vi "PSK_Mod_Transmit_test.vi"() -> ()   [LabVIEW 2014]
uses:
  <vilib>/addons/Modulation/Digital/General/MT Generate Bits (Galois, PN Order).vi
  <vilib>/addons/Modulation/Digital/Support/Common/Validators/mod_Generate Bits Validate.vi
  <vilib>/addons/Modulation/Analog/support/mod_Set Error Source.vi
  <vilib>/addons/Modulation/Digital/General/MT Generate PSK System Parameters(M).vi
  <vilib>/addons/Modulation/Digital/Support/Common/Validators/mod_Generate Filter Coefficients Validate.vi
  <vilib>/addons/Modulation/Digital/General/subVIs/mod_Generate Filter Coefficients.vi
  <vilib>/addons/Modulation/Digital/General/subVIs/mod_Generate Bits PN Sequence.vi
  <vilib>/addons/Modulation/Digital/General/MT Generate PSK Synchronization Parameters (bit array).vi
  <vilib>/addons/Modulation/Digital/General/MT Generate Bits (User Defined).vi
  <instrlib>/niUSRP/niUSRP Write Tx Data (CDB Cluster).vi
  <vilib>/addons/Modulation/niDMT.lvlib
  <vilib>/addons/Modulation/niAMT.lvlib
panel:
  out "Before demod&compensation":waveform(dbl)(graph)
  in  "stop":bool
  in  "error in (no error)":errorcluster
  out "error out":errorcluster
  in  "USRP IP address":refnum<k15>="192.168.10.1"
  in  "Tx Parameters":T1={"Tx IQ Sampling\nRate [s/sec]"=400000.0, "Tx Frequency [Hz]"=5795000000.0, "Tx Gain [dB]"=0.0, "Tx Antenna"="TX1"} {"Tx Gain [dB]" format="%#.6p"; "Tx Frequency [Hz]" format="%#.6p"; "Tx IQ Sampling\nRate [s/sec]" format="%#.6p"}
  out "Actual Tx Parameters":T1={"Tx IQ Sampling\nRate [s/sec]"=400000.0, "Tx Frequency [Hz]"=915000000.0, "Tx Gain [dB]"=0.0, "Tx Antenna"="TX1"} {"Tx Gain [dB]" format="%#.6p"; "Tx Frequency [Hz]" format="%#.6p"; "Tx IQ Sampling\nRate [s/sec]" format="%#.6p"}
  in  "user base bit pattern":i8[](array[numeric]) caption="Input bit stream"
  out "bits sent":i32
  out "Constellation Graph":T2(graph) caption="Tx Signal Constellation"
  out "input bit stream":i8[](array[numeric]) caption="input package"
  in  "filter parameters":T3={"Alpha"=0.5, "Filter Length"=6, "TX Filter"=enum."Root Raised Cos"} {"Alpha" format="%.2f"}
  in  "QPSK System Parameters":T4={"Samples per Symbol"=8, "symbol map"=[], "Differential PSK"=enum."disable", "PSK type"=0} {"PSK type" items=["normal", "shifted", "offset"]; "symbol map" format="%.3f"}
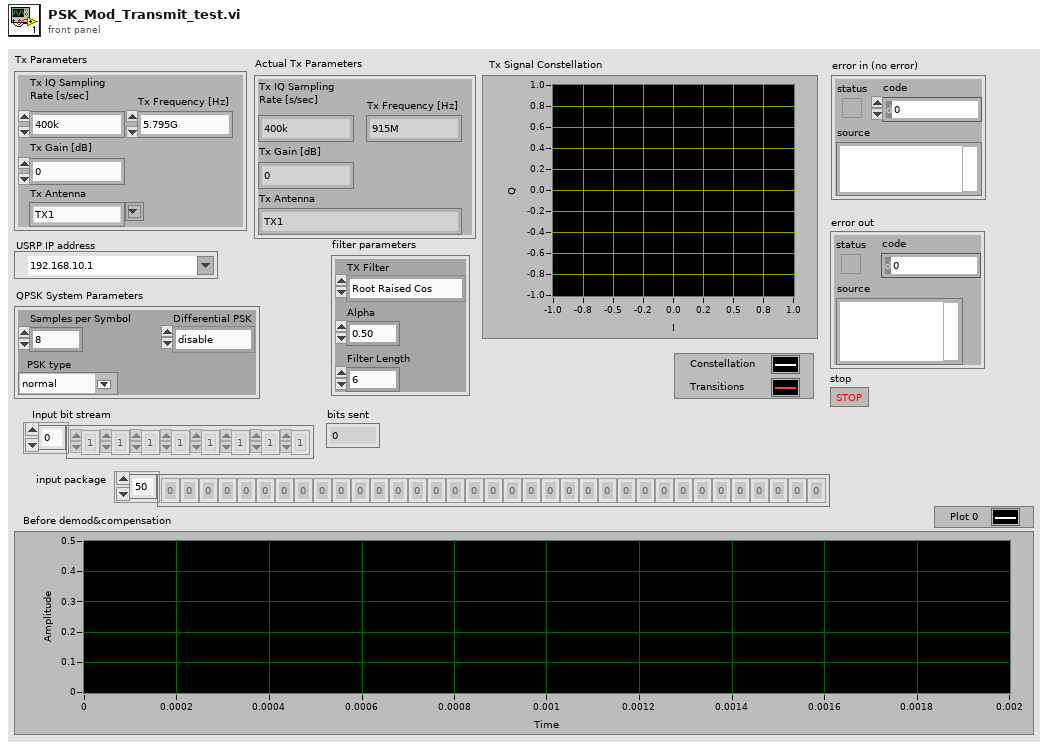
[diagram p1: front panel]
types:
  T1 = cluster{"Tx IQ Sampling\nRate [s/sec]":dbl, "Tx Frequency [Hz]":dbl, "Tx Gain [dB]":dbl, "Tx Antenna":string}
  T2 = cluster{"constellation":dbl[], "oversampled data":dbl[]}[]
  T3 = cluster{"Alpha":dbl, "Filter Length":i32, "TX Filter":enum16{"none", "Raised Cosine", "Root Raised Cos", "Gaussian"}}
  T4 = cluster{"Samples per Symbol":i32, "symbol map":cdb[], "Differential PSK":enum16{"disable", "enable"}, "PSK type":u16}
  T5 = enum16{"FSK", "PSK", "QAM", "MSK", "PAM", "ASK", "CPM"}
  T6 = enum16{"none", "Raised Cosine", "Root Raised Cos", "Gaussian"}
  T7 = cluster{"samples per symbol (16)":i32, "symbol map":cdb[], "differential PSK":enum16{"disable", "enable"}, "PSK type":u16}
  T8 = cluster{"expected sync location (symbols)":i32, "sync sequence":cdb[], "sync location uncertainty (symbols)":i32, "sync indent (symbols)":i32}
  T9 = typedef "niAMT.lvlib/Complex Data Waveform.ctl" = cluster{"t0":dbl, "dt":dbl, "Y":cdb[]}
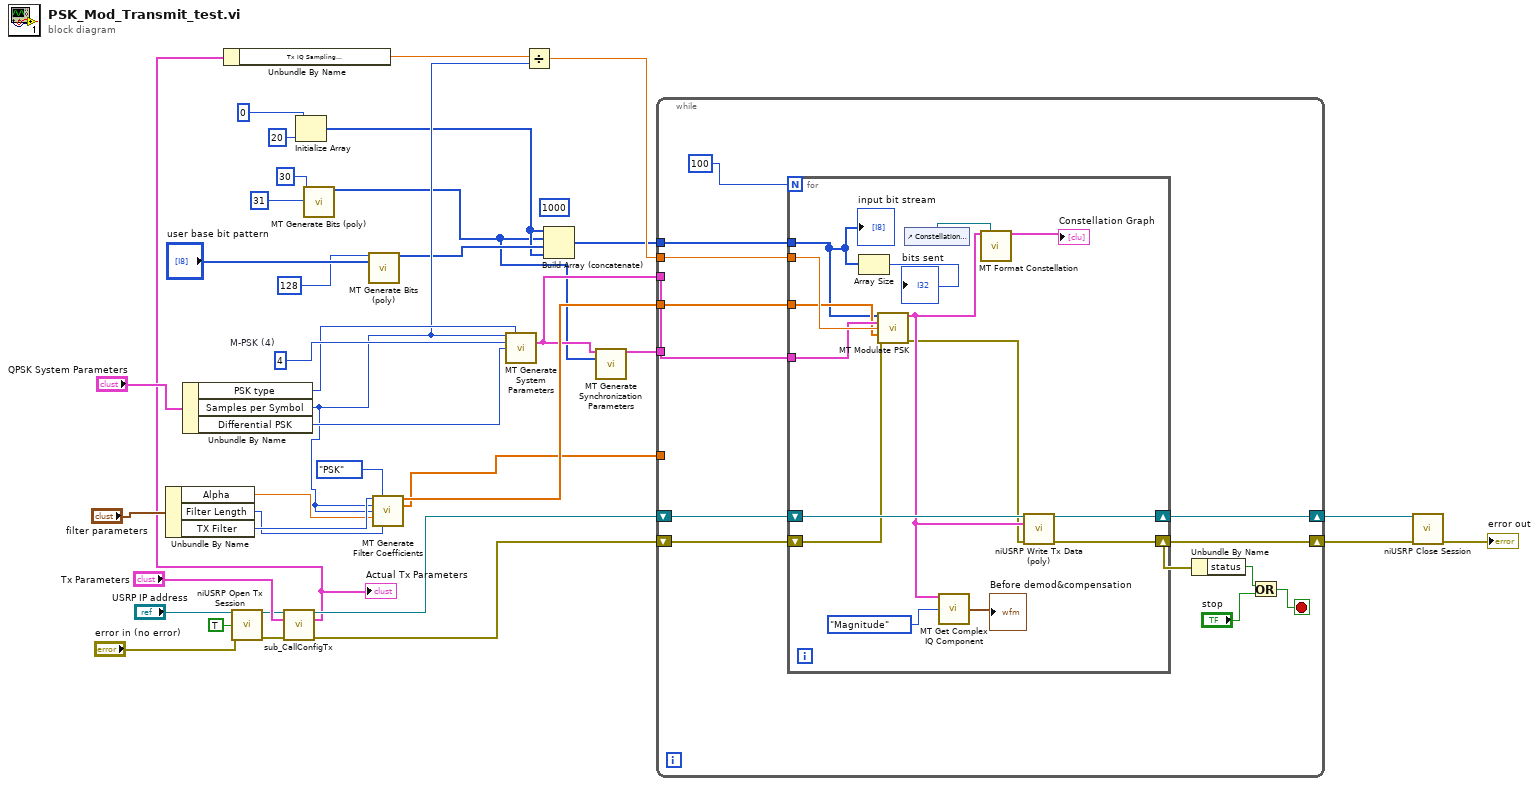
[diagram p0: block diagram]
diagram:
  (unwired) 1000 ("dimension size")
  w36 = 4  # M-PSK (4)
  n1 = Unbundle By Name("filter parameters") -> ("Alpha"=w32:dbl, "Filter Length"=w33:i32, "TX Filter"=w34:T6)
  n2 = Unbundle By Name("QPSK System Parameters") -> ("PSK type"=w35:u16, "Samples per Symbol"=w24:i32, "Differential PSK"=w37:enum16{"disable", "enable"})
  n3 = call <instrlib>:"niUSRP Open Tx Session.vi"("device names"="USRP IP address", "reset"=TRUE, "error in (no error)"="error in (no error)") -> ("session handle out"=w20:refnum<k15>, "error out"=w19:errorcluster)  [unwired: 11 in]
  n4 = call "sub_CallConfigTx.vi"("session handle"=w20, "Tx Parameters"="Tx Parameters", "error in"=w19) -> ("session handle out"=w13:refnum<k15>, "Actual Tx Parameters"=w10:T1, "error out"=w14:errorcluster)  [unwired: 10 in]
  "Actual Tx Parameters" <- w10
  n5 = Unbundle By Name(w10) -> ("Tx IQ Sampling\nRate [s/sec]"=w9:dbl)
  n6 = Initialize Array(i8 0 ("element"), 20 ("dimension size")) -> (w6:i8[])
  n7 = call-poly <vilib>:"MT Generate Bits (poly).vi"("total bits (128)"=30, "PN sequence order (9)"=31) -> ("output bit stream"=w4:i8[])  [unwired: 11 in, 2 out]
  n8 = call-poly <vilib>:"MT Generate Bits (poly).vi"("total bits (128)"=128, "user base bit pattern"="user base bit pattern") -> ("output bit stream"=w23:i8[])  [unwired: 12 in, 1 out]
  n9 = call <vilib>:"MT Generate Filter Coefficients.vi"("pulse shaping filter (none)"=w34, "modulation type"=T5."PSK", "pulse shaping samples per symbol (16)"=w24, "matched samples per symbol (16)"=w24, "filter parameter"=w32, "filter length (symbols)"=w33) -> ("pulse shaping filter coefficients"=w7:dbl[], "matched filter coefficients"=w2:dbl[])  [unwired: 7 in, 1 out]
  n10 = call-poly <vilib>:"MT Generate System Parameters.vi"("samples per symbol (16)"=w24, "PSK type"=w35, "M-PSK (4)"=w36, "differential PSK"=w37) -> ("PSK system parameters"=w5:T7)  [unwired: 9 in, 2 out]
  n11 = Divide(x=w9, y=w24) -> (x/y=w8:dbl)
  n12 = Build Array (concatenate)(w6, w4, w23, w6) -> (w1:i8[])
  n13 = call-poly <vilib>:"MT Generate Synchronization Parameters.vi"("PSK system parameters"=w5, "sync bits"=w4) -> ("PSK synchronization parameters"=w3:T8)  [unwired: 12 in, 1 out]
  n14 = while {
    shift-right: [w43] -> w11
    shift-left: w14 -> [w47]
    shift-right: [w49] -> w12
    shift-left: w13 -> [w50]
    tunnel: w1 -> [w44]
    tunnel: w5 -> [w46]
    tunnel: w8 -> [w48]
    tunnel: w7 -> [w45]
    tunnel: w3 -> [_]
    tunnel: w2 -> [_]
    stop <- w41 stop-if-true
    n15 = for {
      N: 100 -> [_]
      tunnel: w48 -> [w62]
      tunnel: w46 -> [w58]
      tunnel: w45 -> [w57]
      tunnel: w44 -> [w56]
      shift-right: [w64] -> w49
      shift-left: w50 -> [w65]
      shift-right: [w52] -> w43
      shift-left: w47 -> [w61]
      n16 = Array Size(array=w56) -> (size(s)=→"bits sent":i32)
      n17 = call <vilib>:"MT Modulate PSK.vi"("input bit stream"=w56, "PSK system parameters"=w58, "symbol rate (Hz)"=w62, "pulse shaping filter coefficients"=w57, "error in (no error)"=w61) -> ("output complex waveform"=w53:T9, "error out"=w51:errorcluster)  [unwired: 8 in, 1 out]
      n18 = control-ref of="Constellation Graph"() -> (w59:refnum<vi>)
      n19 = call <vilib>:"MT Get Complex IQ Component.vi"("IQ data (complex) in"=w53, "component choice"=enum16{"I", "Q", "Magnitude", "Phase"}."Magnitude") -> ("CE component"=→"Before demod&compensation":waveform(dbl))  [unwired: 11 in, 2 out]
      n20 = call <vilib>:"MT Format Constellation.vi"("waveform"=w53, "constellation reference"=w59) -> ("constellation graph"=→"Constellation Graph":T2)  [unwired: 12 in, 1 out]
      n21 = call-poly <instrlib>:"niUSRP Write Tx Data (poly).vi"("session handle"=w65, "data"=w53, "error in (no error)"=w51) -> ("session handle out"=w64:refnum<k15>, "error out"=w52:errorcluster)  [unwired: 11 in]
      "input bit stream" <- w56
    }
    n22 = Unbundle By Name(w43) -> ("status"=w42:bool)
    n23 = Or(x=w42, y="stop") -> (x .or. y?=w41:bool)
  }
  n24 = call <instrlib>:"niUSRP Close Session.vi"("session handle"=w12, "error in (no error)"=w11) -> ("error out"=→"error out":errorcluster)  [unwired: 13 in]
